vi "Unregister for Stimulus Profile Session Undeploy Event.vi"(8 "error in (no error)":errorcluster, 11 "Session Undeploy Event Ref":T1) -> (0 "error out":errorcluster)   [LabVIEW 2020, in "NI_VS Sequence Execution Interface.lvlib"]
doc: "Unregisters for a session undeploy event. Use the Register for Stimulus Profile Session Undeploy Event VI to get the <B>Session Undeploy Event Ref</B> this VI expects."
uses:
  <vilib>/NI VeriStand/Execution/SequenceExecutionInterface/NI_VS Sequence Execution Interface.lvlib
  <vilib>/NI VeriStand/Execution/SequenceExecutionInterface/Session Event Ref.ctl
  <vilib>/NI VeriStand/Execution/SequenceExecutionInterface/Stimulus Profile Session Ref.ctl
  NationalInstruments.VeriStand.ClientAPI
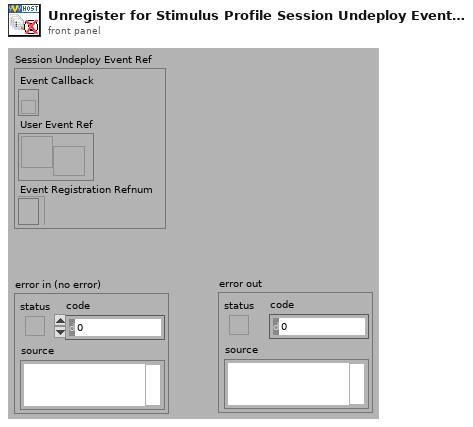
[diagram p1: front panel]
types:
  T1 = typedef "NI_VS Sequence Execution Interface.lvlib/Session Event Ref.ctl" = cluster{"Event Callback":refnum<k27>, "User Event Ref":refnum<user-event>, "Event Registration Refnum":refnum<event-registration>}
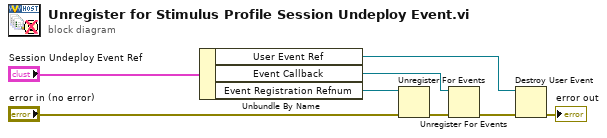
[diagram p0: block diagram]
diagram:
  n1 = Unbundle By Name("Session Undeploy Event Ref") -> ("User Event Ref"=w2:refnum<user-event>, "Event Callback"=w5:refnum<k27>, "Event Registration Refnum"=w7:refnum<event-registration>)
  n2 = Unregister For Events(event registration refnum=w7, error in="error in (no error)") -> (error out=w4:errorcluster)
  n3 = Unregister For Events(event registration refnum=w5, error in=w4) -> (error out=w3:errorcluster)
  n4 = Destroy User Event(user event=w2, error in=w3) -> (error out=→"error out":errorcluster)
